vi "[FGV] CaliperEntry.vi"(6 "CoordSystemRun":bool=TRUE, 7 "Action":T6, 8 "error in (no error)":errorcluster, 11 "CaliperEntriesIn":T1[](array[typedef]) {"CaliperType" items=["Distance", "Mid Point", "Perpendicular Projection", "Lines Intersection", "Angle from Horizontal", "Angle from Vertical", "Angle Defined by 3 Points", "Angle Defined by 4 Points", "Bissecting Line", "Mid Line", "Center of Mass", "Area", "Line Fit", "Circle Fit", "Ellipse Fit"]}) -> (0 "error out":errorcluster, 3 "AllCaliperEntries":T1[](array[typedef]) {"CaliperType" items=["Distance", "Mid Point", "Perpendicular Projection", "Lines Intersection", "Angle from Horizontal", "Angle from Vertical", "Angle Defined by 3 Points", "Angle Defined by 4 Points", "Bissecting Line", "Mid Line", "Center of Mass", "Area", "Line Fit", "Circle Fit", "Ellipse Fit"]})   [LabVIEW 2019]
uses:
  Controls/Caliper_Entry_FGV_Action.ctl
  Controls/CaliperDataEntry.ctl
  Controls/CaliperType.ctl
  Controls/SelectionListEntry.ctl
  Controls/SelectionListEntryPointType.ctl
  Controls/CaliperResult.ctl
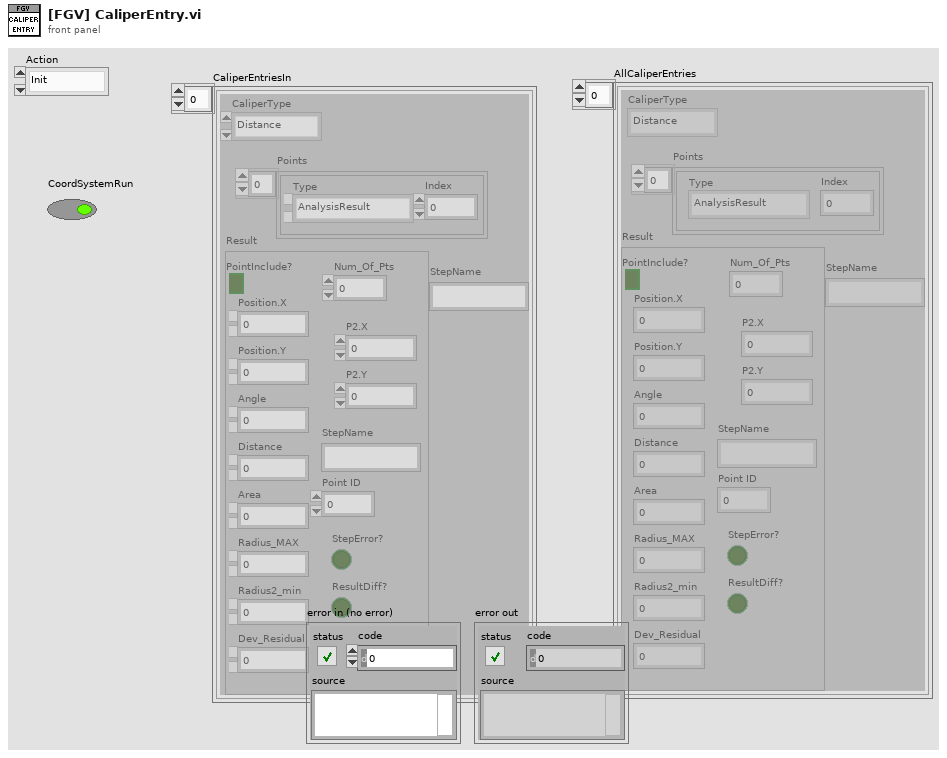
[diagram p1: front panel]
types:
  T1 = typedef "CaliperDataEntry.ctl" = cluster{"CaliperType":T2, "Points":T3[], "Result":T5, "StepName":string}
  T2 = typedef "CaliperType.ctl" = u32
  T3 = typedef "SelectionListEntry.ctl" = cluster{"Type":T4, "Index":i32}
  T4 = typedef "SelectionListEntryPointType.ctl" = enum16{"AnalysisResult", "CaliperResult"}
  T5 = typedef "CaliperResult.ctl" = cluster{"PointInclude?":bool, "Num_Of_Pts":u8, "Position.X":dbl, "Position.Y":dbl, "Angle":dbl, "Distance":dbl, "Area":dbl, "Radius_MAX":dbl, "Radius2_min":dbl, "Dev_Residual":dbl, "P2.X":dbl, "P2.Y":dbl, "StepName":string, "Point ID":u8, "StepError?":bool, "ResultDiff?":bool}
  T6 = typedef "Caliper_Entry_FGV_Action.ctl" = enum16{"Init", "Close", "Add", "Delete", "ReplaceAll", "ReadAll"}
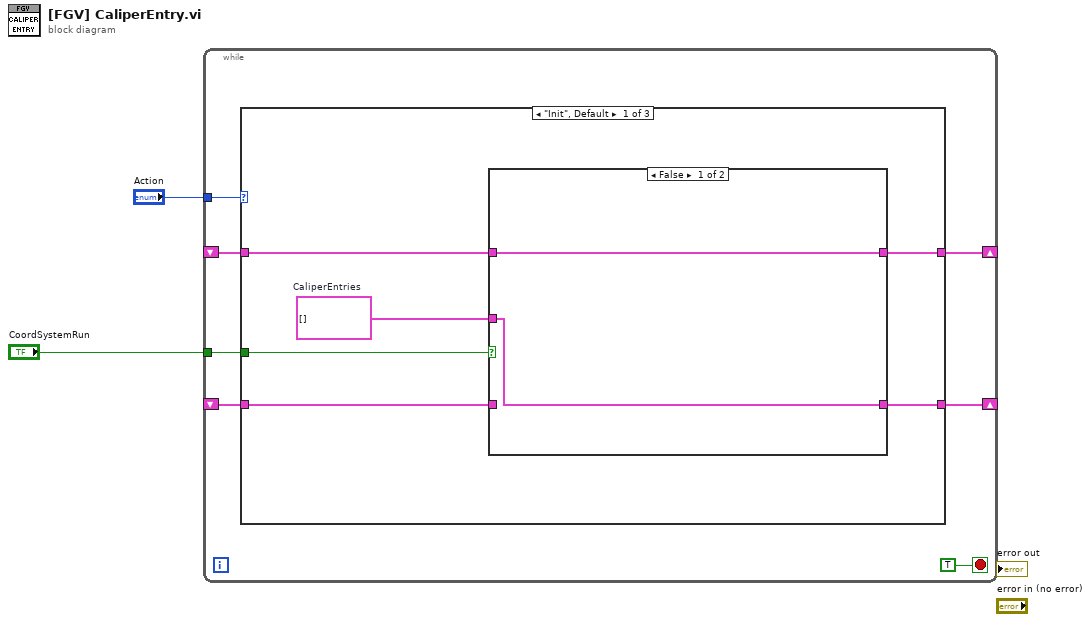
[diagram p0: block diagram]
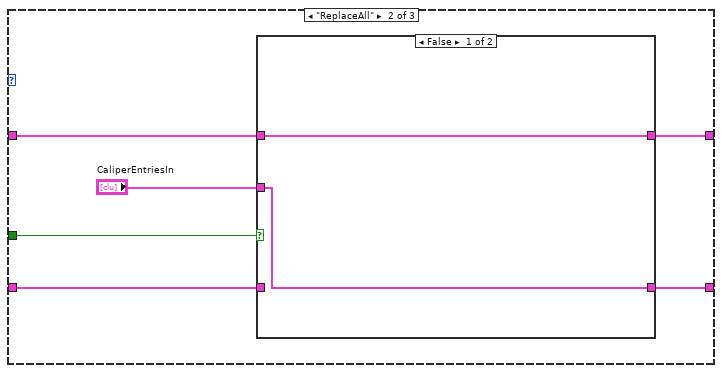
[diagram p3: hidden frame]
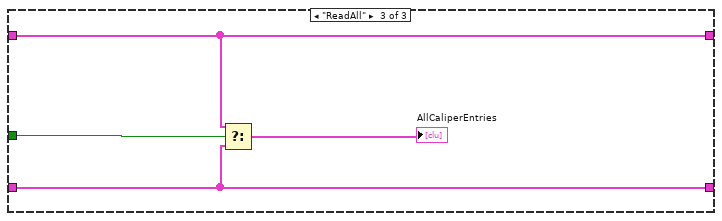
[diagram p5: hidden frame]
diagram:
  n1 = while {
    tunnel: "Action" -> [w8]
    shift-right: [w7] -> _
    shift-left: _ -> [w6]
    tunnel: "CoordSystemRun" -> [w5]
    shift-right: [w4] -> _
    shift-left: _ -> [w3]
    stop <- TRUE stop-if-true
    n2 = case shown="\"Init\", Default" w8 {
      tunnel: [w11 w19 w31] -> w7
      tunnel: w6 -> [w15 w21 w31]
      tunnel: w5 -> [w14 w24 w32]
      tunnel: [w10 w22 w29] -> w4
      tunnel: w3 -> [w13 w23 w29]
      frame "Init", Default {
        w12 = T1[] []  # CaliperEntries
        n3 = case shown="False" w14 {
          tunnel: w15 -> [w17 _]
          tunnel: w13 -> [_ _]
          tunnel: w12 -> [w16 w18]
          tunnel: [w17 w18] -> w11
          tunnel: [w16 w18] -> w10
          frame False {
          }
          frame True {
          }
        }
      }
      frame "ReplaceAll" {
        n4 = case shown="False" w24 {
          tunnel: w23 -> [_ w28]
          tunnel: [w25 w28] -> w22
          tunnel: w21 -> [w26 _]
          tunnel: "CaliperEntriesIn" -> [w25 w27]
          tunnel: [w26 w27] -> w19
          frame False {
          }
          frame True {
          }
        }
      }
      frame "ReadAll" {
        n5 = Select(t=w31, s=w32, f=w29) -> (s? t:f=→"AllCaliperEntries":T1[])
      }
    }
  }
